vi "Blynk Heartbeat.vi"(8 "error in":errorcluster, 11 "connection":refnum<k5>) -> (0 "error out":errorcluster, 3 "connection out":refnum<k5>)   [LabVIEW 2014]
uses:
  utilities/MsgType.ctl
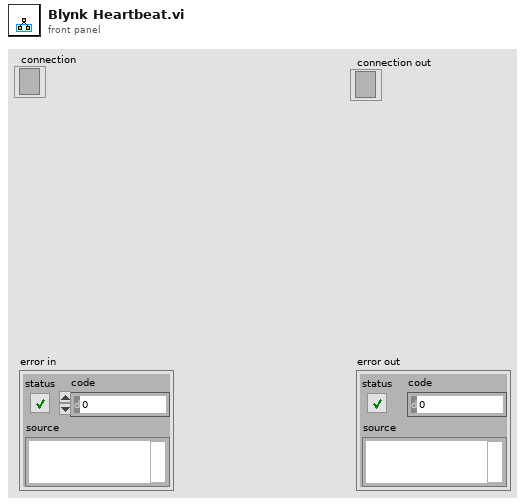
[diagram p1: front panel]
types:
  T1 = typedef "MsgType.ctl" = enum8{"RSP", "REGISTER", "LOGIN", "SAVE_PROF", "LOAD_PROF", "GET_TOKEN", "PING", "ACTIVATE", "DEACTIVATE", "REFRESH", "UNDEFINED0", "UNDEFINED1", "TWEET", "EMAIL", "NOTIFY", "BRIDGE", "UNDEFINED2", "UNDEFINED3", "UNDEFINED4", "UNDEFINED5", "HW"}
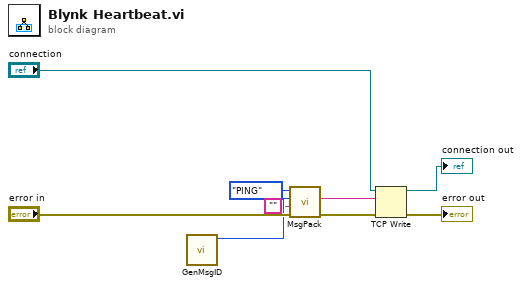
[diagram p0: block diagram]
diagram:
  n1 = call "GenMsgID.vi"() -> ("MsgID"=w3:u16)  [unwired: 10 in, 1 out]
  n2 = call "MsgPack.vi"("error in"="error in", "msg"="", "msg_id"=w3, "msg_type"=MsgType."PING") -> ("error out"=w8:errorcluster, "msg_data"=w2:string)  [unwired: 6 in]
  n3 = TCP Write(connection ID="connection", data in=w2, error in (no error)=w8) -> (connection ID out=→"connection out":refnum<k5>, error out=→"error out":errorcluster)  [unwired: 1 in, 1 out]
